vi "System-Plot-Host.vi"() -> ()   [LabVIEW 2016]
uses:
  Shared/Typedefs/System-QuickIDsArray.ctl
  <vilib>/addons/Software Calibration Management/xSCM/Controls/ID and Element.ctl
  <vilib>/addons/Software Calibration Management/XControls/TBL1D.xctl
  <vilib>/addons/Software Calibration Management/XControls/TBL2D.xctl
  Shared/DSI-Shared.lvlib
  <vilib>/addons/Software Calibration Management/xSCM/SCM-API.lvlib
panel:
  in  "SYS|Plot|Universal":sgl[][](array[numeric])
  in  "SYS|Plot|Units":string[](array[string])
  in  "SYS|Plot|Names":string[](array[string])
  in  "SYS|Plot|Max":sgl[](array[numeric])
  in  "SYS|Plot|Min":sgl[](array[numeric])
  out "SYS|Plot|Dims":u8
  out "SYS|Plot|Variant":variant
  in  "_Modify.B":bool
  in  "_Chart.B":bool
  out "SYS|Plot|Unit":string caption="Units"
  in  "SYS|Plot|Select":u8
  out "SYS|Plot|Values":sgl[](array[numeric])
  in  "_Refresh":bool
  in  "SYS|Plot|IDs":T1
  out "SYS|Plot|Type":T3(ring)
  in  "_ModeTabs":enum32{"Chart", "Universal", "1DTBL", "2DTBL"}(tab)
  out "_Chart":T4(graph)
  in  "_Table":string[][](table)
  in  "SYS|Plot|1DTLU":cluster{"X":sgl[], "Y":sgl[]}(xcontrol)
  in  "SYS|Plot|2DTLU":cluster{"X":sgl[], "Y":sgl[], "Z":sgl[][]}(xcontrol)
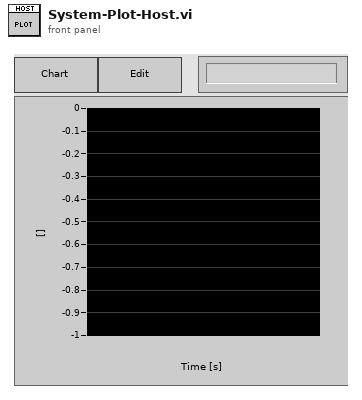
[diagram p1: front panel]
types:
  T1 = typedef "DSI-Shared.lvlib/System-QuickIDsArray.ctl" = T2[]
  T2 = typedef "SCM-API.lvlib/ID and Element.ctl" = cluster{"ID":u32, "Element":i32[]}
  T3 = enum8{"BOL", "U8", "U16", "U32", "U64", "I8", "I16", "I32", "I64", "SGL", "DBL", "EXT", "CSG", "CDB", "CXT", "STR", "TBL", "TLU", "CTM"}
  T4 = cluster{"[0]":sgl, "[1]":sgl, "[2]":sgl, "[3]":sgl, "[4]":sgl, "[5]":sgl, "[6]":sgl, "[7]":sgl, "[8]":sgl, "[9]":sgl, "[10]":sgl, "[11]":sgl, "[12]":sgl, "[13]":sgl, "[14]":sgl, "[15]":sgl, "[16]":sgl, "[17]":sgl, "[18]":sgl, "[19]":sgl, "[20]":sgl, "[21]":sgl, "[22]":sgl, "[23]":sgl, "[24]":sgl, "[25]":sgl, "[26]":sgl, "[27]":sgl, "[28]":sgl, "[29]":sgl, "[30]":sgl, "[31]":sgl, "[32]":sgl, "[33]":sgl, "[34]":sgl, "[35]":sgl, "[36]":sgl, "[37]":sgl, "[38]":sgl, "[39]":sgl, "[40]":sgl, "[41]":sgl, "[42]":sgl, "[43]":sgl, "[44]":sgl, "[45]":sgl, "[46]":sgl, "[47]":sgl, "[48]":sgl, "[49]":sgl, "[50]":sgl, "[51]":sgl, "[52]":sgl, "[53]":sgl, "[54]":sgl, "[55]":sgl, "[56]":sgl, "[57]":sgl, "[58]":sgl, "[59]":sgl, "[60]":sgl, "[61]":sgl, "[62]":sgl, "[63]":sgl, "[64]":sgl, "[65]":sgl, "[66]":sgl, "[67]":sgl, "[68]":sgl, "[69]":sgl, "[70]":sgl, "[71]":sgl, "[72]":sgl, "[73]":sgl, "[74]":sgl, "[75]":sgl, "[76]":sgl, "[77]":sgl, "[78]":sgl, "[79]":sgl, "[80]":sgl, "[81]":sgl, "[82]":sgl, "[83]":sgl, "[84]":sgl, "[85]":sgl, "[86]":sgl, "[87]":sgl, "[88]":sgl, "[89]":sgl, "[90]":sgl, "[91]":sgl, "[92]":sgl, "[93]":sgl, "[94]":sgl, "[95]":sgl, "[96]":sgl, "[97]":sgl, "[98]":sgl, "[99]":sgl}
  T5 = enum8{"Enabled", "Disabled", "Disabled and Grayed Out"}
  T6 = enum32{"Invalid", "Standard", "Closed", "Hidden", "Minimized", "Maximized"}
  T7 = cluster{"SYS|Plot|Values[0]":sgl, "SYS|Plot|Values[1]":sgl, "SYS|Plot|Values[2]":sgl, "SYS|Plot|Values[3]":sgl, "SYS|Plot|Values[4]":sgl, "SYS|Plot|Values[5]":sgl, "SYS|Plot|Values[6]":sgl, "SYS|Plot|Values[7]":sgl, "SYS|Plot|Values[8]":sgl, "SYS|Plot|Values[9]":sgl, "SYS|Plot|Values[10]":sgl, "SYS|Plot|Values[11]":sgl, "SYS|Plot|Values[12]":sgl, "SYS|Plot|Values[13]":sgl, "SYS|Plot|Values[14]":sgl, "SYS|Plot|Values[15]":sgl, "SYS|Plot|Values[16]":sgl, "SYS|Plot|Values[17]":sgl, "SYS|Plot|Values[18]":sgl, "SYS|Plot|Values[19]":sgl, "SYS|Plot|Values[20]":sgl, "SYS|Plot|Values[21]":sgl, "SYS|Plot|Values[22]":sgl, "SYS|Plot|Values[23]":sgl, "SYS|Plot|Values[24]":sgl, "SYS|Plot|Values[25]":sgl, "SYS|Plot|Values[26]":sgl, "SYS|Plot|Values[27]":sgl, "SYS|Plot|Values[28]":sgl, "SYS|Plot|Values[29]":sgl, "SYS|Plot|Values[30]":sgl, "SYS|Plot|Values[31]":sgl, "SYS|Plot|Values[32]":sgl, "SYS|Plot|Values[33]":sgl, "SYS|Plot|Values[34]":sgl, "SYS|Plot|Values[35]":sgl, "SYS|Plot|Values[36]":sgl, "SYS|Plot|Values[37]":sgl, "SYS|Plot|Values[38]":sgl, "SYS|Plot|Values[39]":sgl, "SYS|Plot|Values[40]":sgl, "SYS|Plot|Values[41]":sgl, "SYS|Plot|Values[42]":sgl, "SYS|Plot|Values[43]":sgl, "SYS|Plot|Values[44]":sgl, "SYS|Plot|Values[45]":sgl, "SYS|Plot|Values[46]":sgl, "SYS|Plot|Values[47]":sgl, "SYS|Plot|Values[48]":sgl, "SYS|Plot|Values[49]":sgl, "SYS|Plot|Values[50]":sgl, "SYS|Plot|Values[51]":sgl, "SYS|Plot|Values[52]":sgl, "SYS|Plot|Values[53]":sgl, "SYS|Plot|Values[54]":sgl, "SYS|Plot|Values[55]":sgl, "SYS|Plot|Values[56]":sgl, "SYS|Plot|Values[57]":sgl, "SYS|Plot|Values[58]":sgl, "SYS|Plot|Values[59]":sgl, "SYS|Plot|Values[60]":sgl, "SYS|Plot|Values[61]":sgl, "SYS|Plot|Values[62]":sgl, "SYS|Plot|Values[63]":sgl, "SYS|Plot|Values[64]":sgl, "SYS|Plot|Values[65]":sgl, "SYS|Plot|Values[66]":sgl, "SYS|Plot|Values[67]":sgl, "SYS|Plot|Values[68]":sgl, "SYS|Plot|Values[69]":sgl, "SYS|Plot|Values[70]":sgl, "SYS|Plot|Values[71]":sgl, "SYS|Plot|Values[72]":sgl, "SYS|Plot|Values[73]":sgl, "SYS|Plot|Values[74]":sgl, "SYS|Plot|Values[75]":sgl, "SYS|Plot|Values[76]":sgl, "SYS|Plot|Values[77]":sgl, "SYS|Plot|Values[78]":sgl, "SYS|Plot|Values[79]":sgl, "SYS|Plot|Values[80]":sgl, "SYS|Plot|Values[81]":sgl, "SYS|Plot|Values[82]":sgl, "SYS|Plot|Values[83]":sgl, "SYS|Plot|Values[84]":sgl, "SYS|Plot|Values[85]":sgl, "SYS|Plot|Values[86]":sgl, "SYS|Plot|Values[87]":sgl, "SYS|Plot|Values[88]":sgl, "SYS|Plot|Values[89]":sgl, "SYS|Plot|Values[90]":sgl, "SYS|Plot|Values[91]":sgl, "SYS|Plot|Values[92]":sgl, "SYS|Plot|Values[93]":sgl, "SYS|Plot|Values[94]":sgl, "SYS|Plot|Values[95]":sgl, "SYS|Plot|Values[96]":sgl, "SYS|Plot|Values[97]":sgl, "SYS|Plot|Values[98]":sgl, "SYS|Plot|Values[99]":sgl}
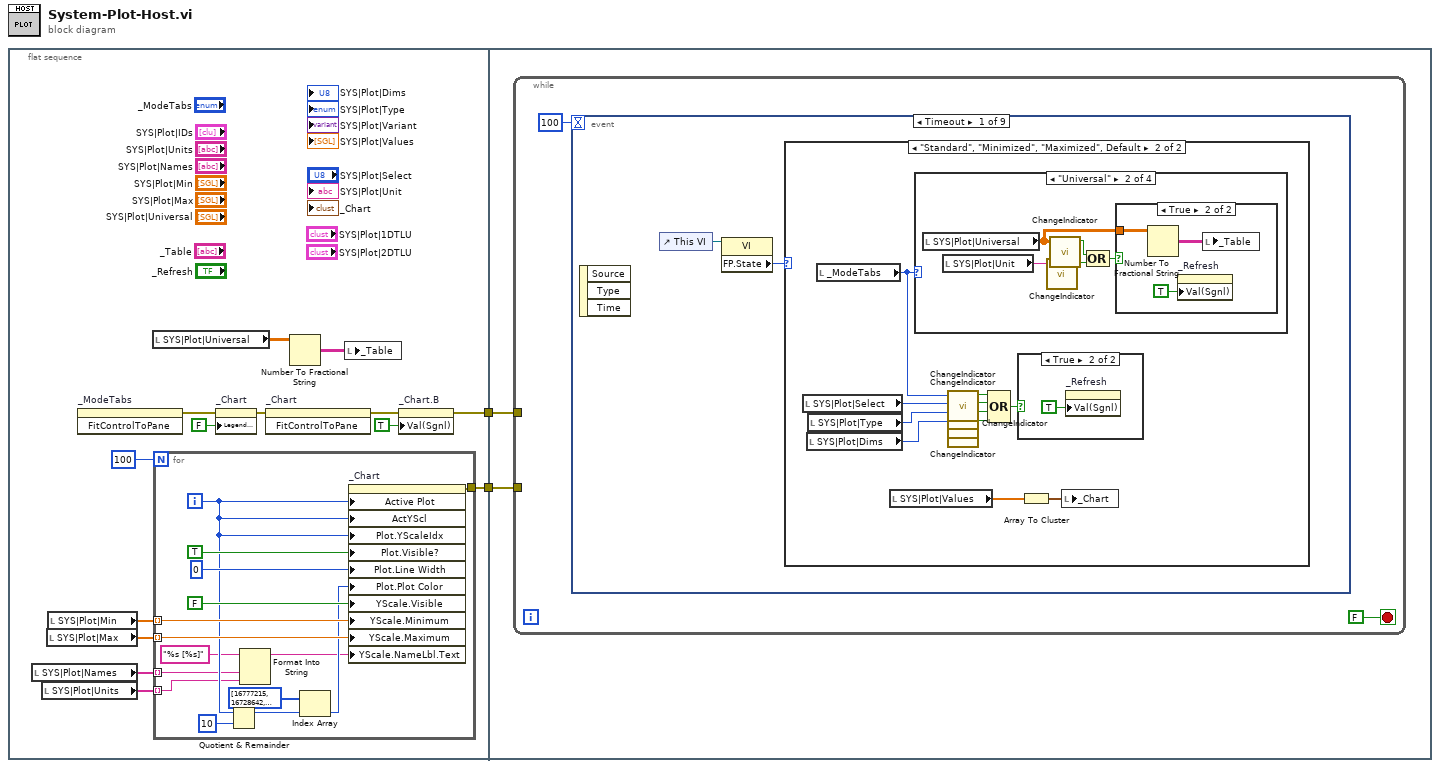
[diagram p0: block diagram]
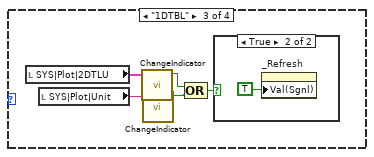
[diagram p6: hidden frame]
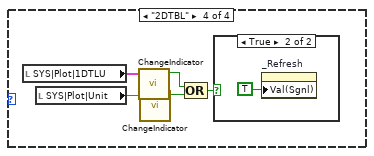
[diagram p8: hidden frame]
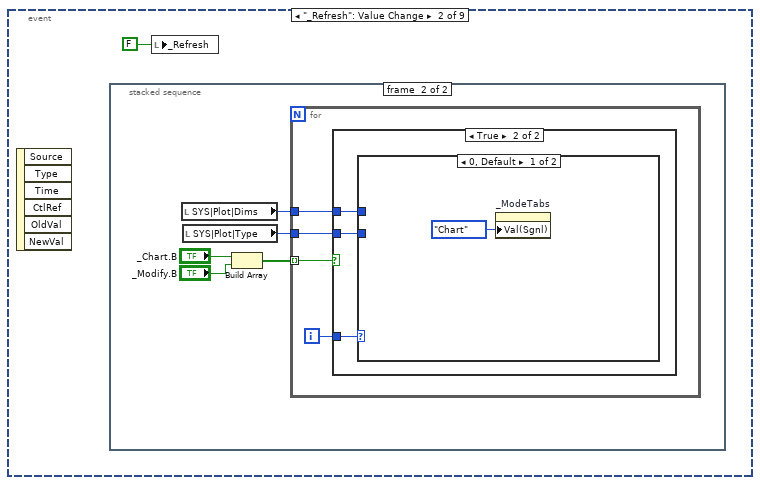
[diagram p10: hidden frame]
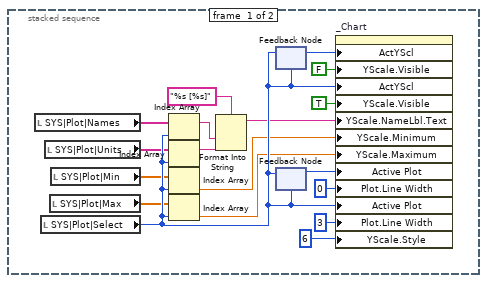
[diagram p11: hidden frame]
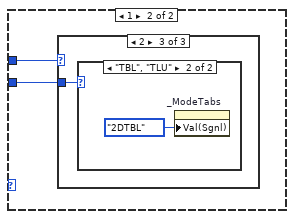
[diagram p13: hidden frame]
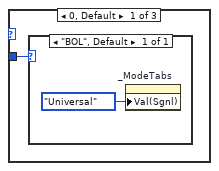
[diagram p14: hidden frame]
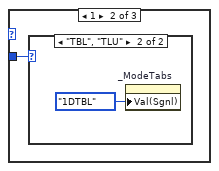
[diagram p15: hidden frame]
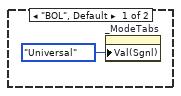
[diagram p16: hidden frame]
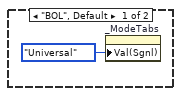
[diagram p17: hidden frame]
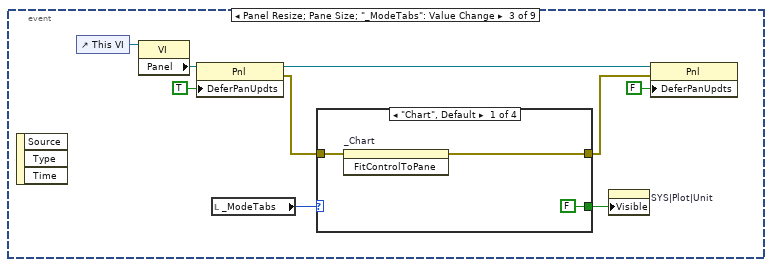
[diagram p18: hidden frame]
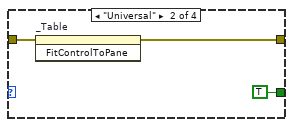
[diagram p19: hidden frame]
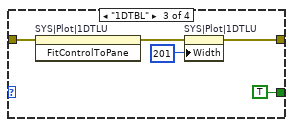
[diagram p20: hidden frame]
diagram:
  n1 = flat-sequence {
    tunnel: [w5] -> w2
    tunnel: [w15] -> w1
    tunnel: w2 -> [w33]
    tunnel: w1 -> [w32]
    frame #0 {
      n2 = local read "SYS|Plot|Names"() -> (w9:string[])
      n3 = local read "SYS|Plot|Units"() -> (w8:string[])
      n4 = local read "SYS|Plot|Max"() -> (w10:sgl[])
      n5 = local read "SYS|Plot|Min"() -> (w11:sgl[])
      n6 = invoke on="_ModeTabs" class="TabCtl (strict)" method="FitControlToPane"() -> (error out=w14:errorcluster)  [unwired: 3 in, 2 out]
      n7 = local read "SYS|Plot|Universal"() -> (w3:sgl[][])
      n8 = for {
        N: 100 -> [_]
        tunnel: [w26] -> w15
        tunnel: w11 -> [w28] mode=indexing
        tunnel: w10 -> [w27] mode=indexing
        tunnel: w9 -> [w18] mode=indexing
        tunnel: w8 -> [w17] mode=indexing
        i -> [w23]
        n9 = Quotient & Remainder(x=w23, y=10) -> (x-y*floor(x/y)=w21:i32)  [unwired: 1 out]
        n10 = Format Into String(format string="%s [%s]", w18, w17) -> (resulting string=w19:string)  [unwired: 2 in, 1 out]
        n11 = Index Array(array=u32[] [16777215, 16728642, 982784, 4375295, 13827953, 13457919, 16757522, 4343295, 16728758, 5898228] ("Array"), index=w21) -> (element=w24:u32)
        n12 = property on="_Chart" class="WFChart (strict)"("Active Plot"=w23, "ActYScl"=w23, "Plot.YScaleIdx"=w23, "Plot.Visible?"=TRUE ("Plot.Visible"), "Plot.Line Width"=u8 0, "Plot.Plot Color"=w24, "YScale.Visible"=FALSE ("Y Scale.Visible"), "YScale.Minimum"=w28, "YScale.Maximum"=w27, "YScale.NameLbl.Text"=w19) -> (error out=w26:errorcluster)  [unwired: 2 in, 1 out]
      }
      n13 = property on="_Chart" class="WFChart (strict)"(error in=w14, "Legend Visible"=FALSE ("Legend:Visible")) -> (error out=w13:errorcluster)  [unwired: 1 in, 1 out]
      n14 = invoke on="_Chart" class="WFChart (strict)" method="FitControlToPane"(error in=w13) -> (error out=w6:errorcluster)  [unwired: 2 in, 2 out]
      n15 = Number To Fractional String(number=w3) -> (F-format string=w4:string[][])  [unwired: 3 in]
      n16 = local write "_Table"(w4) -> ()
      n17 = property on="_Chart.B" class="Bool (strict)"(error in=w6, "Val(Sgnl)"=TRUE ("Value (Signaling)")) -> (error out=w5:errorcluster)  [unwired: 1 in, 1 out]
    }
    frame #1 {
      n18 = while {
        tunnel: w33 -> [_]
        tunnel: w32 -> [_]
        stop <- FALSE stop-if-true
        n19 = event shown="[0] Timeout" {
          selector: _ -> [_ _ _ _ _ _ _ _ _]
          dyn-events: _ -> [_ _ _ _ _ _ _ _ _]
          timeout: 100 -> [_ _ _ _ _ _ _ _ _]
          event Timeout {
            n20 = event-data() -> ()  [unwired: 1 in, 3 out]
            n21 = control-ref of="This VI"() -> (w37:refnum<vi>)
            n22 = property class="VI"(reference=w37) -> ("FP.State"=w36:T6)  [unwired: 1 in, 2 out]
            n23 = case shown="\"Standard\", \"Minimized\", \"Maximized\", Default" w36 {
              frame "Invalid", "Closed", "Hidden" {
              }
              frame "Standard", "Minimized", "Maximized", Default {
                n24 = local read "SYS|Plot|Select"() -> (w45:u8)
                n25 = local read "SYS|Plot|Dims"() -> (w38:u8)
                n26 = local read "SYS|Plot|Type"() -> (w41:T3)
                n27 = local read "_ModeTabs"() -> (w47:enum32{"Chart", "Universal", "1DTBL", "2DTBL"})
                n28 = local read "SYS|Plot|Values"() -> (w46:sgl[])
                n29 = case shown="\"Universal\"" w47 {
                  frame "Chart", Default {
                  }
                  frame "Universal" {
                    n30 = local read "SYS|Plot|Universal"() -> (w50:sgl[][])
                    n31 = local read "SYS|Plot|Unit"() -> (w54:string)
                    n32 = call "ChangeIndicator.vi"("Input"=w54) -> ("Change"=w52:bool)  [unwired: 9 in]
                    n33 = call "ChangeIndicator.vi"("Input"=w50) -> ("Change"=w53:bool)  [unwired: 9 in]
                    n34 = Compound Arithmetic op=OR(w53, w52) -> (w51:bool)
                    n35 = case shown="True" w51 {
                      tunnel: w50 -> [_ w55]
                      frame False {
                      }
                      frame True {
                        n36 = Number To Fractional String(number=w55) -> (F-format string=w56:string[][])  [unwired: 3 in]
                        n37 = property on="_Refresh" class="Bool (strict)"("Val(Sgnl)"=TRUE ("Value (Signaling)")) -> ()  [unwired: 2 in, 2 out]
                        n38 = local write "_Table"(w56) -> ()
                      }
                    }
                  }
                  frame "1DTBL" {
                    n39 = local read "SYS|Plot|2DTLU"() -> (w62:cluster{"X":sgl[], "Y":sgl[], "Z":sgl[][]})
                    n40 = local read "SYS|Plot|Unit"() -> (w61:string)
                    n41 = call "ChangeIndicator.vi"("Input"=w62) -> ("Change"=w60:bool)  [unwired: 9 in]
                    n42 = call "ChangeIndicator.vi"("Input"=w61) -> ("Change"=w59:bool)  [unwired: 9 in]
                    n43 = Compound Arithmetic op=OR(w60, w59) -> (w58:bool)
                    n44 = case shown="True" w58 {
                      frame False {
                      }
                      frame True {
                        n45 = property on="_Refresh" class="Bool (strict)"("Val(Sgnl)"=TRUE ("Value (Signaling)")) -> ()  [unwired: 2 in, 2 out]
                      }
                    }
                  }
                  frame "2DTBL" {
                    n46 = local read "SYS|Plot|1DTLU"() -> (w68:cluster{"X":sgl[], "Y":sgl[]})
                    n47 = local read "SYS|Plot|Unit"() -> (w67:string)
                    n48 = call "ChangeIndicator.vi"("Input"=w68) -> ("Change"=w66:bool)  [unwired: 9 in]
                    n49 = call "ChangeIndicator.vi"("Input"=w67) -> ("Change"=w65:bool)  [unwired: 9 in]
                    n50 = Compound Arithmetic op=OR(w66, w65) -> (w64:bool)
                    n51 = case shown="True" w64 {
                      frame False {
                      }
                      frame True {
                        n52 = property on="_Refresh" class="Bool (strict)"("Val(Sgnl)"=TRUE ("Value (Signaling)")) -> ()  [unwired: 2 in, 2 out]
                      }
                    }
                  }
                }
                n53 = call "ChangeIndicator.vi"("Input"=w47) -> ("Change"=w44:bool)  [unwired: 9 in]
                n54 = call "ChangeIndicator.vi"("Input"=w45) -> ("Change"=w43:bool)  [unwired: 9 in]
                n55 = call "ChangeIndicator.vi"("Input"=w41) -> ("Change"=w40:bool)  [unwired: 9 in]
                n56 = call "ChangeIndicator.vi"("Input"=w38) -> ("Change"=w39:bool)  [unwired: 9 in]
                n57 = Compound Arithmetic op=OR(w44, w43, w40, w39) -> (w42:bool)
                n58 = case shown="True" w42 {
                  frame False {
                  }
                  frame True {
                    n59 = property on="_Refresh" class="Bool (strict)"("Val(Sgnl)"=TRUE ("Value (Signaling)")) -> ()  [unwired: 2 in, 2 out]
                  }
                }
                n60 = Array To Cluster(array=w46) -> (cluster=w48:T7)
                n61 = local write "_Chart"(w48) -> ()
              }
            }
          }
          event "_Refresh": Value Change {
            n62 = event-data() -> ()  [unwired: 1 in, 6 out]
            n63 = stacked-sequence {
              frame #0 {
                n64 = local read "SYS|Plot|Names"() -> (w71:string[])
                n65 = local read "SYS|Plot|Select"() -> (w86:u8)
                n66 = local read "SYS|Plot|Units"() -> (w72:string[])
                n67 = local read "SYS|Plot|Max"() -> (w77:sgl[])
                n68 = local read "SYS|Plot|Min"() -> (w78:sgl[])
                n69 = Index Array(array=w71, index=w86) -> (element=w74:string)
                n70 = Index Array(array=w72, index=w86) -> (element=w73:string)
                n71 = Index Array(array=w78, index=w86) -> (element=w79:sgl)
                n72 = Index Array(array=w77, index=w86) -> (element=w80:sgl)
                n73 = Format Into String(format string="%s [%s]", w74, w73) -> (resulting string=w76:string)  [unwired: 2 in, 1 out]
                n74 = feedback #1(w86) -> (w85:u8)
                n75 = feedback-in #1(w86) -> ()
                n76 = feedback #2(w86) -> (w83:u8)
                n77 = feedback-in #2(w86) -> ()
                n78 = property on="_Chart" class="WFChart (strict)"("ActYScl"=w85, "YScale.Visible"=FALSE ("Y Scale.Visible"), "ActYScl"=w86, "YScale.Visible"=TRUE ("Y Scale.Visible"), "YScale.NameLbl.Text"=w76, "YScale.Minimum"=w79, "YScale.Maximum"=w80, "Active Plot"=w83, "Plot.Line Width"=u8 0, "Active Plot"=w86, "Plot.Line Width"=u8 3, "YScale.Style"=u8 6 ("Y Scale.Style")) -> ()  [unwired: 2 in, 2 out]
              }
              frame #1 {
                n79 = local read "SYS|Plot|Dims"() -> (w93:u8)
                n80 = local read "SYS|Plot|Type"() -> (w92:T3)
                n81 = Build Array("_Chart.B", "_Modify.B") -> (w91:bool[])
                n82 = for {
                  tunnel: w91 -> [w97] mode=indexing
                  tunnel: w92 -> [w95]
                  tunnel: w93 -> [w94]
                  i -> [w96]
                  n83 = case shown="True" w97 {
                    tunnel: w96 -> [_ w100]
                    tunnel: w95 -> [_ w99]
                    tunnel: w94 -> [_ w98]
                    frame False {
                    }
                    frame True {
                      n84 = case shown="0, Default" w100 {
                        tunnel: w99 -> [_ w102]
                        tunnel: w98 -> [_ w103]
                        frame 0, Default {
                          n85 = property on="_ModeTabs" class="TabCtl (strict)"("Val(Sgnl)"=enum32{"Chart", "Universal", "1DTBL", "2DTBL"}."Chart" ("Value (Signaling)")) -> ()  [unwired: 2 in, 2 out]
                        }
                        frame 1 {
                          n86 = case shown="2" w103 {
                            tunnel: w102 -> [w104 w106 w109]
                            frame 0, Default {
                              n87 = case shown="\"BOL\", Default" w104 {
                                frame "BOL", Default {
                                n88 = property on="_ModeTabs" class="TabCtl (strict)"("Val(Sgnl)"=enum32{"Chart", "Universal", "1DTBL", "2DTBL"}."Universal" ("Value (Signaling)")) -> ()  [unwired: 2 in, 2 out]
                                }
                              }
                            }
                            frame 1 {
                              n89 = case shown="\"TBL\", \"TLU\"" w106 {
                                frame "BOL", Default {
                                n90 = property on="_ModeTabs" class="TabCtl (strict)"("Val(Sgnl)"=enum32{"Chart", "Universal", "1DTBL", "2DTBL"}."Universal" ("Value (Signaling)")) -> ()  [unwired: 2 in, 2 out]
                                }
                                frame "TBL", "TLU" {
                                n91 = property on="_ModeTabs" class="TabCtl (strict)"("Val(Sgnl)"=enum32{"Chart", "Universal", "1DTBL", "2DTBL"}."1DTBL" ("Value (Signaling)")) -> ()  [unwired: 2 in, 2 out]
                                }
                              }
                            }
                            frame 2 {
                              n92 = case shown="\"TBL\", \"TLU\"" w109 {
                                frame "BOL", Default {
                                n93 = property on="_ModeTabs" class="TabCtl (strict)"("Val(Sgnl)"=enum32{"Chart", "Universal", "1DTBL", "2DTBL"}."Universal" ("Value (Signaling)")) -> ()  [unwired: 2 in, 2 out]
                                }
                                frame "TBL", "TLU" {
                                n94 = property on="_ModeTabs" class="TabCtl (strict)"("Val(Sgnl)"=enum32{"Chart", "Universal", "1DTBL", "2DTBL"}."2DTBL" ("Value (Signaling)")) -> ()  [unwired: 2 in, 2 out]
                                }
                              }
                            }
                          }
                        }
                      }
                    }
                  }
                }
              }
            }
            n95 = local write "_Refresh"(FALSE ("_Refresh")) -> ()
          }
          event Panel Resize; Pane Size; "_ModeTabs": Value Change {
            n96 = event-data() -> ()  [unwired: 1 in, 3 out]
            n97 = control-ref of="This VI"() -> (w115:refnum<vi>)
            n98 = property class="VI"(reference=w115) -> ("Panel"=w116:refnum<vi>)  [unwired: 1 in, 2 out]
            n99 = property class="Pnl"(reference=w116, "DeferPanUpdts"=TRUE ("Defer Panel Updates")) -> (reference out=w119:refnum<vi>, error out=w114:errorcluster)  [unwired: 1 in]
            n100 = local read "_ModeTabs"() -> (w120:enum32{"Chart", "Universal", "1DTBL", "2DTBL"})
            n101 = case shown="\"Chart\", Default" w120 {
              tunnel: w114 -> [w123 w126 w129 w134]
              tunnel: [w122 w125 w128 w133] -> w113
              tunnel: [FALSE ("Defer Panel Updates") TRUE ("Defer Panel Updates") TRUE ("Defer Panel Updates") TRUE ("Defer Panel Updates")] -> w112
              frame "Chart", Default {
                n102 = invoke on="_Chart" class="WFChart (strict)" method="FitControlToPane"(error in=w123) -> (error out=w122:errorcluster)  [unwired: 2 in, 2 out]
              }
              frame "Universal" {
                n103 = invoke on="_Table" class="Tbl (strict)" method="FitControlToPane"(error in=w126) -> (error out=w125:errorcluster)  [unwired: 2 in, 2 out]
              }
              frame "1DTBL" {
                n104 = invoke on="SYS|Plot|1DTLU" class="TBL1D (strict)" method="FitControlToPane"(error in=w129) -> (error out=w130:errorcluster)  [unwired: 2 in, 2 out]
                n105 = property on="SYS|Plot|1DTLU" class="TBL1D (strict)"(error in=w130, "Width"=u32 201 ("XControl:Container Bounds:Width")) -> (error out=w128:errorcluster)  [unwired: 1 in, 1 out]
              }
              frame "2DTBL" {
                n106 = invoke on="SYS|Plot|2DTLU" class="TBL2D (strict)" method="FitControlToPane"(error in=w134) -> (error out=w133:errorcluster)  [unwired: 2 in, 2 out]
              }
            }
            n107 = property on="SYS|Plot|Unit" class="Str"("Visible"=w112) -> ()  [unwired: 2 in, 2 out]
            n108 = property class="Pnl"(reference=w119, error in=w113, "DeferPanUpdts"=FALSE ("Defer Panel Updates")) -> ()  [unwired: 2 out]
          }
          event "_Chart": Scale Range Change {
            w138 = 100 ("dimension size")
            n109 = event-data() -> ()  [unwired: 1 in, 8 out]
            n110 = local read "SYS|Plot|Select"() -> (w135:u8)
            n111 = local read "SYS|Plot|Min"() -> (w144:sgl[])
            n112 = local read "SYS|Plot|Max"() -> (w143:sgl[])
            n113 = property on="_Chart" class="WFChart (strict)"("ActYScl"=w135) -> ("YScale.Minimum"=w142:dbl, "YScale.Maximum"=w141:dbl)  [unwired: 2 in, 2 out]
            n114 = Reshape Array(w144, w138) -> (w140:sgl[])
            n115 = Reshape Array(w143, w138) -> (w139:sgl[])
            n116 = Replace Array Subset(array=w140, new element=w142, index=w135) -> (w137:sgl[])
            n117 = Replace Array Subset(array=w139, new element=w141, index=w135) -> (w136:sgl[])
            n118 = property on="SYS|Plot|Min" class="Arr (strict)"("Val(Sgnl)"=w137) -> ()  [unwired: 2 in, 2 out]
            n119 = property on="SYS|Plot|Max" class="Arr (strict)"("Val(Sgnl)"=w136) -> ()  [unwired: 2 in, 2 out]
          }
          event "_Chart.B", "_Modify.B": Value Change {
            n120 = event-data() -> ("CtlRef"=w153:refnum<vi>)  [unwired: 1 in]
            n121 = feedback #3(w153) -> (w147:refnum<vi>)
            n122 = feedback-in #3(w153) -> ()
            n123 = property class="Bool (strict)"(reference=w147, "Value"=FALSE, "DisabledEnum"=T5."Enabled" ("Disabled")) -> (error out=w152:errorcluster)  [unwired: 1 in, 1 out]
            n124 = property class="Bool (strict)"(reference=w153, error in=w152, "Value"=TRUE, "DisabledEnum"=T5."Disabled" ("Disabled")) -> (error out=w145:errorcluster)  [unwired: 1 out]
            n125 = property on="_Refresh" class="Bool (strict)"(error in=w145, "Val(Sgnl)"=TRUE ("Value (Signaling)")) -> ()  [unwired: 1 in, 2 out]
          }
          event "_Table": Value Change {
            n126 = event-data() -> ("NewVal"=w157:string[][])  [unwired: 1 in]
            n127 = Fract/Exp String To Number(string=w157) -> (number=w156:dbl[][])  [unwired: 3 in, 1 out]
            n128 = local read "SYS|Plot|Dims"() -> (w158:u8)
            n129 = case shown="0, Default" w158 {
              tunnel: w156 -> [w163 w166 w167]
              tunnel: [w159 w164 w167] -> w155
              frame 0, Default {
                w160 = 0 ("index (row)")
                n130 = Index Array(array=w163, index (row)=w160, index (col)=w160) -> (element=w162:dbl)
                n131 = Build Array(w162) -> (w161:dbl[])
                n132 = Build Array(w161) -> (w159:dbl[][])
              }
              frame 1 {
                n133 = Index Array(array=w166) -> (element=w165:dbl[])  [unwired: 2 in]
                n134 = Build Array(w165) -> (w164:dbl[][])
              }
              frame 2 {
              }
            }
            n135 = Number To Fractional String(number=w155) -> (F-format string=w154:string[][])  [unwired: 3 in]
            n136 = property on="SYS|Plot|Universal" class="Arr (strict)"("Val(Sgnl)"=w155) -> ()  [unwired: 2 in, 2 out]
            n137 = property on="_Table" class="Tbl (strict)"("Value"=w154) -> ()  [unwired: 2 in, 2 out]
          }
          event "SYS|Plot|1DTLU", "SYS|Plot|2DTLU": Shortcut Menu Activation? {
            n138 = event-data() -> ("MenuRef"=w171:refnum<k9>)  [unwired: 1 in, 1 out]
            n139 = Insert Menu Items(7:"APP_SEPARATOR" ("item tags"), 8:"-" ("item names"), 9:w171) -> (3:w170:refnum<k9>)  [unwired: 3 in, 2 out]
            n140 = Insert Menu Items(7:"_RESIZE" ("item tags"), 8:"Resize Table", 9:w170) -> ()  [unwired: 3 in, 3 out]
            n141 = event-data() -> ()  [unwired: 2 in, 1 out]
          }
          event "SYS|Plot|1DTLU": Shortcut Menu Selection (User) {
            n142 = event-data() -> ("ItemTag"=w174:string)  [unwired: 1 in]
            n143 = case shown="\"_RESIZE\"" w174 {
              frame Default {
              }
              frame "_RESIZE" {
                n144 = control-ref of="SYS|Plot|1DTLU"() -> (w175:refnum<vi>)
                n145 = call "Resize Table 1D.vi"("1D Table"=w175) -> ()  [unwired: 11 in]
              }
            }
          }
          event "SYS|Plot|2DTLU": Shortcut Menu Selection (User) {
            n146 = event-data() -> ("ItemTag"=w176:string)  [unwired: 1 in, 1 out]
            n147 = case shown="\"_RESIZE\"" w176 {
              frame Default {
              }
              frame "_RESIZE" {
                n148 = control-ref of="SYS|Plot|2DTLU"() -> (w177:refnum<vi>)
                n149 = call "Resize Table 2D.vi"("2D Table"=w177) -> ()  [unwired: 11 in]
              }
            }
          }
        }
      }
    }
  }
